vi "Basic.vi"() -> ()   [LabVIEW 2022 SP3, in "GettingStarted_5774_Host.lvlib"]
uses:
  GettingStarted_5774_Host.lvlib
  <vilib>/userDefined/High Color/nirio_resource_hc.ctl
  <instrlib>/FlexRIO/API/Host/v1/NI FlexRIO/API/Reference Clock Source.ctl
  <vilib>/FPGAPlugInAG/PXIe-5774 (KU060)/niLvFpga_Open_PXIe-5774 (KU060).vi
  <vilib>/rvi/interface/common/dynamic/niFpgaDynamicAddResources.vi
  <instrlib>/FlexRIO/API/Host/v1/NI FlexRIO/API/Configure Reference Clock.vi
  <instrlib>/FlexRIO/API/Host/v1/NI FlexRIO/API/Get Property Reference - Fpga Small.vi
  <instrlib>/FlexRIO/API/Host/v1/NI FlexRIO/API/Configure Analog Start Trigger.vi
  <instrlib>/FlexRIO/API/Host/v1/NI FlexRIO/API/Configure Digital Edge Start Trigger.vi
  <instrlib>/FlexRIO/API/Host/v1/NI FlexRIO/API/Configure Immediate Start Trigger.vi
  <instrlib>/FlexRIO/API/Host/v1/NI FlexRIO/API/Read Stream 1D WDT.vi
  <vilib>/measure/maspectr.llb/FFT Power Spectrum and PSD for N Chan.vi
  <vilib>/Utility/error.llb/Error Cluster From Error Code.vi
  <vilib>/rvi/errors/niLvFpgaAdjustHostInterfaceError.vi
  <vilib>/FPGAPlugInAG/Dynamic/niLvFpga_Close_Dynamic.vi
  <vilib>/rvi/interface/nirviOpenFPGA/nirviOpenFPGA.xnode
  FPGA Bitfiles/PXIe_5774_KU060.lvbitx
  <vilib>/rvi/interface/nirviReadWriteControl/nirviReadWriteControl.xnode
  <vilib>/rvi/interface/nirviCloseFPGA/nirviCloseFPGA.xnode
  <instrlib>/FlexRIO/API/Host/v1/NI FlexRIO API v1.lvlib
  <resource>/objmgr/niflexrioapiStream.rc
  <vilib>/measure/NI_MAPro.lvlib
  <resource>/objmgr/niflexrioapiChannel.rc
  NiFpgaLv.dll
  <vilib>/rvi/interface/Simulation/niFpgaSimulationCallBeginRW.vi
panel:
  in  "Threshold":i16
  out "HighValue":bool
  in  "reference clock source":T1 items=["Default", "Onboard", "PXI_Clk10", "External", "None", "Baseboard Reference"]
  in  "AI1 Range":dbl(ring)=1.0 items=["1V"=1.0, "200mV"=0.2]
  in  "AI0 Range":dbl(ring)=1.0 items=["1V"=1.0, "200mV"=0.2]
  in  "AI1 Offset (V)":dbl
  in  "AI0 Offset (V)":dbl
  out "Sample Rate":dbl=3200000000.0 format="%#_6p"
  in  "ADC Interleaving Factor":i32=1 min=0 max=2 step=1
  in  "AI num samples":u64=320 step=16
  in  "AI channels":string="AI0,AI1"
  out "Device Power":dbl(slide) scale=-1.0..38.0 scale format="%#_3p"
  out "FPGA Temperature":dbl(slide) scale=0.0..100.0 scale format="%#_3p"
  in  "Trigger Type":enum32{"Immediate", "Analog", "Digital"}(tab)
  in  "trigger channel":string(combo)="AI0"
  in  "rising edge?":bool=TRUE
  in  "level (V)":dbl format="%#_3p"
  in  "hysteresis (V)":dbl format="%#_3p"
  in  "digital trigger source":string(combo)
  in  "stop":bool
  in  "Waveform Tab Control":enum32{"AI Time Domain", "AI Frequency Domain"}(tab)
  out "Waveform Graph":waveform(dbl)[](graph)
  out "FFT":cluster{"f0":dbl, "df":dbl, "magnitude":dbl[]}[](graph) caption="Waveform Graph"
  out "error out":errorcluster
  out "Limit (W)":dbl
  out "Power (W)":dbl
  out "Limit (C)":dbl
  out "Temp (C)":dbl format="%#_4p"
  in  "RIO Device":T2
  # "Overview: Configure an acquisition for a FlexRIO target and transfer the data to the host using the FlexRIO Host API.  Loop an output waveform\nRequirements: FlexRIO\nInstructions: \n 1. Select the RIO Device that corresponds to the FlexRIO target. \n 2. Optionally configure the clocking, stream, and trigger. \n 3. Run the VI"
  # "Resource Configuration"
  # "Clocking configuration"
  # "Input Waveform Configuration"
  # "Device Monitoring"
  # "Modified:\nDevice Utilization\n---------------------------\nTotal Slices: 41.3% (17139 out of 41460)\nSlice Registers: 15.5% (102931 out of 663360)\nSlice LUTs: 25.5% (84631 out of 331680)\nBlock RAMs: 23.0% (248 out of 1080)\nDSP48s: 0.2% (6 out of 2760)"
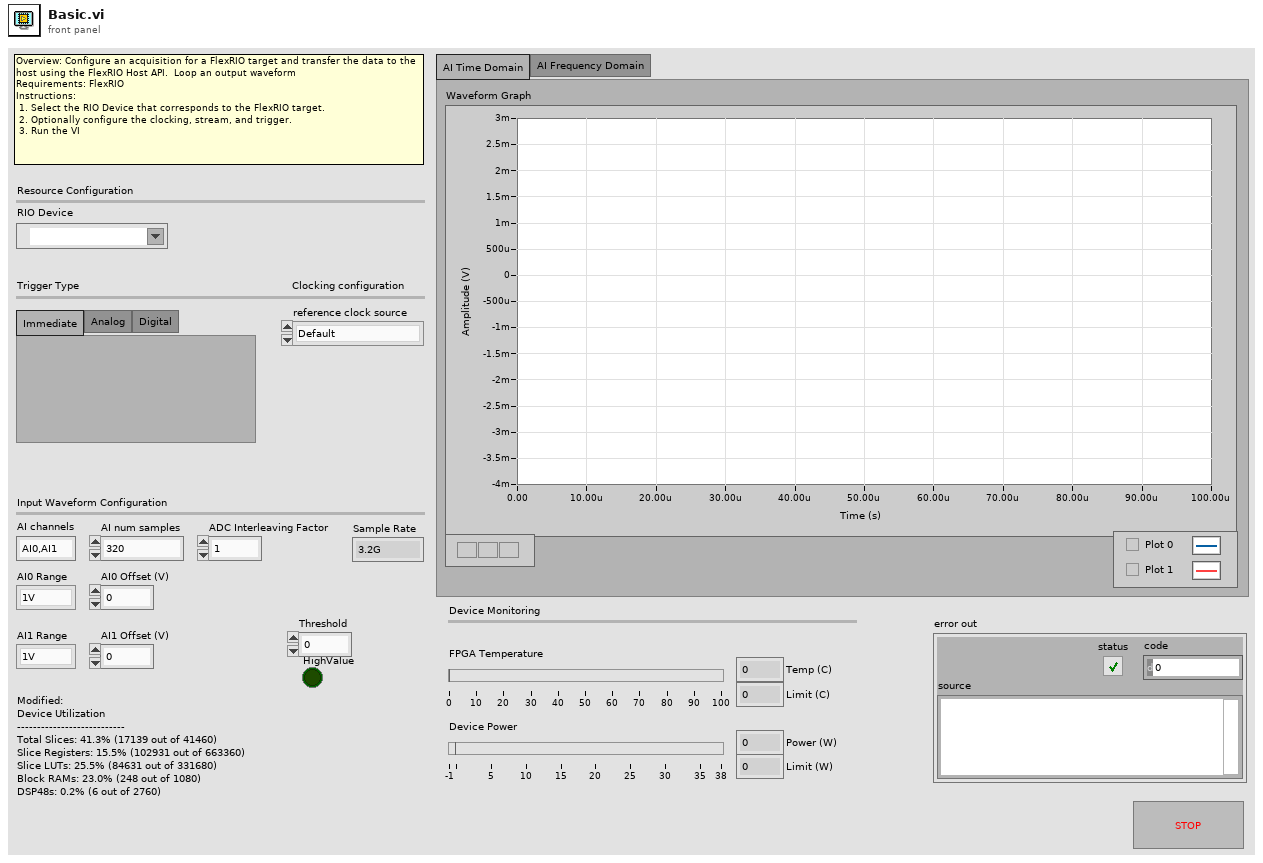
[diagram p1: front panel]
types:
  T1 = typedef "NI FlexRIO API v1.lvlib/Reference Clock Source.ctl" = i32
  T2 = typedef "nirio_resource_hc.ctl" = tag
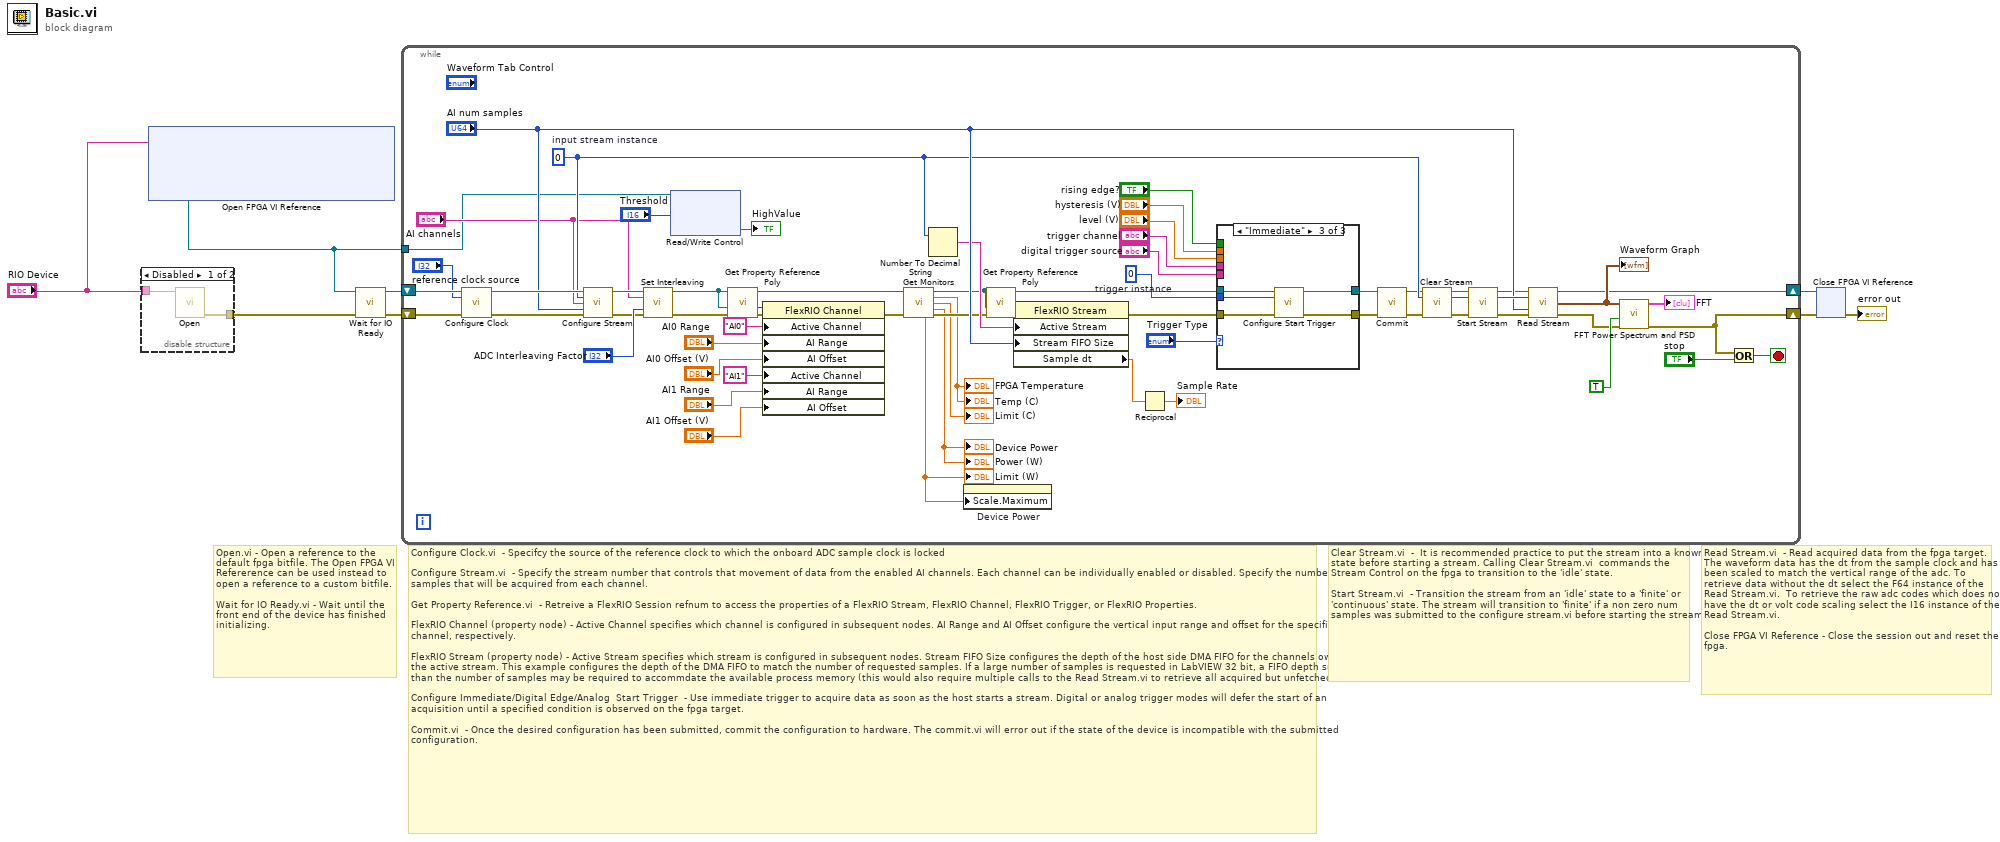
[diagram p0: block diagram]
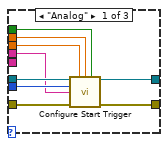
[diagram p3: hidden frame]
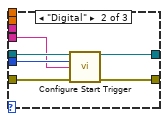
[diagram p4: hidden frame]
diagram:
  # "Read Stream.vi  - Read acquired data from the fpga target. The waveform data has the dt from the sample clock and has been scaled to match the vertical range of the adc. To retrieve data without the dt select the F64 instance of the Read Stream.vi.  To retrieve the raw adc codes which does not have the dt or volt code scaling select the I16 instance of the Read Stream.vi.  \n\nClose FPGA VI Reference - Close the session out and reset the fpga."
  # "Clear Stream.vi  -  It is recommended practice to put the stream into a known state before starting a stream. Calling Clear Stream.vi  commands the Stream Control on the fpga to transition to the 'idle' state.\n\nStart Stream.vi  - Transition the stream from an 'idle' state to a 'finite' or 'continuous' state. The stream will transition to 'finite' if a non zero num samples was submitted to the configure stream.vi before starting the stream."
  # "Configure Clock.vi  - Specifcy the source of the reference clock to which the onboard ADC sample clock is locked\n\nConfigure Stream.vi  - Specify the stream number that controls that movement of data from the enabled AI channels. Each channel can be individually enabled or disabled. Specify the number of samples that will be acquired from each channel. \n\nGet Property Reference.vi  - Retreive a FlexRIO Session refnum to access the properties of a FlexRIO Stream, FlexRIO Channel, FlexRIO Trigger, or FlexRIO Properties.\n\nFlexRIO Channel (property node) - Active Channel specifies which channel is configured in subsequent nodes. AI Range and AI Offset configure the vertical input range and offset for the specified channel, respectively.\n\nFlexRIO Stream (property node) - Active Stream specifies which stream is configured in subsequent nodes. Stream FIFO Size configures the depth of the host side DMA FIFO for the channels owned by the active stream. This example configures the depth of the DMA FIFO to match the number of requested samples. If a large number of samples is requested in LabVIEW 32 bit, a FIFO depth smaller than the number of samples may be required to accommdate the available process memory (this would also require multiple calls to the Read Stream.vi to retrieve all acquired but unfetched data). \n\nConfigure Immediate/Digital Edge/Analog  Start Trigger  - Use immediate trigger to acquire data as soon as the host starts a stream. Digital or analog trigger modes will defer the start of an acquisition until a specified condition is observed on the fpga target. \n\nCommit.vi  - Once the desired configuration has been submitted, commit the configuration to hardware. The commit.vi will error out if the state of the device is incompatible with the submitted configuration."
  # "Open.vi - Open a reference to the default fpga bitfile. The Open FPGA VI Refererence can be used instead to open a reference to a custom bitfile.\n\nWait for IO Ready.vi - Wait until the front end of the device has finished initializing."
  n1 = disable-structure shown="Disabled" {
    disable-tunnel: [w10 _] -> w5
    disable-tunnel: "RIO Device" -> [w9 _]
    frame Disabled {
      n2 = call <instrlib>:"Open.vi"("RIO Device"=w9) -> ("error out"=w10:errorcluster)  [unwired: 13 in, 1 out]
    }
    frame Enabled {
    }
  }
  n3 = xnode "Open FPGA VI Reference"("resource name"="RIO Device") -> ("FPGA VI Reference Out"=w1:refnum<k20>)  [unwired: 1 in, 1 out]
  n4 = call <instrlib>:"Wait for IO Ready.vi"("fpga interface in"=w1, "error in"=w5) -> ("fpga interface out"=w6:refnum<k20>, "error out"=w7:errorcluster)  [unwired: 10 in, 2 out]
  n5 = while {
    shift-right: [w43] -> w3
    shift-left: w7 -> [w58]
    shift-right: [w49] -> w4
    shift-left: w6 -> [w57]
    tunnel: w1 -> [w13]
    stop <- w45 stop-if-true
    w59 = u32 0  # trigger instance
    w48 = u32 0  # input stream instance
    n6 = call-poly <instrlib>:"Configure Clock.vi"("fpga interface in"=w57, "reference clock source"="reference clock source", "error in"=w58) -> ("fpga interface out"=w65:refnum<k20>, "error out"=w64:errorcluster)  [unwired: 11 in]
    n7 = call <instrlib>:"Configure Stream.vi"("fpga interface in"=w65, "stream instance"=w48, "channels enabled"="AI channels", "num samples"="AI num samples", "error in"=w64) -> ("fpga interface out"=w41:refnum<k20>, "error out"=w40:errorcluster)  [unwired: 7 in, 2 out]
    n8 = call "Set Interleaving.vi"("fpga interface in"=w41, "AI channels enabled"="AI channels", "ADC Interleaving Factor"="ADC Interleaving Factor", "error in (no error)"=w40) -> ("fpga interface out"=w15:refnum<k20>, "error out"=w19:errorcluster)  [unwired: 10 in]
    n9 = xnode "Read/Write Control"("FPGA VI Reference In"=w13, "Threshold"="Threshold") -> ("HighValue"=→"HighValue":bool)  [unwired: 1 in, 2 out]
    n10 = call-poly <instrlib>:"Get Property Reference Poly.vi"("error in (no error)"=w19, "fpga interface in"=w15) -> ("error out"=w22:errorcluster, "property reference"=w23:refnum<k20>)  [unwired: 4 in, 1 out]
    n11 = property class="FlexRIO Channel"(reference=w23, error in=w22, "Active Channel"="AI0" ("Active Stream"), "AI Range"="AI0 Range", "AI Offset"="AI0 Offset (V)", "Active Channel"="AI1" ("Active Stream"), "AI Range"="AI1 Range", "AI Offset"="AI1 Offset (V)") -> (error out=w18:errorcluster)  [unwired: 1 out]
    n12 = call "Get Monitors.vi"("fpga interface in"=w15, "error in (no error)"=w18) -> ("fpga interface out"=w36:refnum<k20>, "FPGA Temperature (C)"=→"Temp (C)" →"FPGA Temperature":dbl, "Temperature Limit (C)"=→"Limit (C)":dbl, "Total Power (W)"=→"Power (W)" →"Device Power":dbl, "Power Limit (W)"=w32:dbl, "error out"=w39:errorcluster)  [unwired: 8 in]
    "Limit (W)" <- w32
    n13 = Number To Decimal String(number=w48) -> (decimal integer string=w61:string)  [unwired: 1 in]
    n14 = property on="Device Power" class="Slide (strict)"("Scale.Maximum"=w32) -> ()  [unwired: 2 in, 2 out]
    n15 = call-poly <instrlib>:"Get Property Reference Poly.vi"("error in (no error)"=w39, "fpga interface in"=w36) -> ("error out"=w38:errorcluster, "property reference"=w37:refnum<k20>)  [unwired: 4 in, 1 out]
    n16 = property class="FlexRIO Stream"(reference=w37, error in=w38, "Active Stream"=w61, "Stream FIFO Size"="AI num samples") -> (error out=w52:errorcluster, "Sample dt"=w47:dbl)  [unwired: 1 out]
    n17 = Reciprocal(x=w47) -> (1/x=→"Sample Rate":dbl)
    n18 = case shown="\"Immediate\"" "Trigger Type" {
      tunnel: w36 -> [w81 w87 w92]
      tunnel: w52 -> [w80 w86 w91]
      tunnel: [w79 w85 w90] -> w29
      tunnel: [w78 w84 w89] -> w30
      tunnel: w59 -> [w77 w83 w88]
      tunnel: "trigger channel" -> [w76 _ _]
      tunnel: "level (V)" -> [w75 _ _]
      tunnel: "hysteresis (V)" -> [w74 _ _]
      tunnel: "rising edge?" -> [w73 _ _]
      tunnel: "digital trigger source" -> [_ w82 _]
      frame "Analog" {
        n19 = call-poly <instrlib>:"Configure Start Trigger.vi"("fpga interface in"=w81, "level"=w75, "hysteresis"=w74, "rising edge?"=w73, "trigger instance"=w77, "channel"=w76, "error in"=w80) -> ("fpga interface out"=w79:refnum<k20>, "error out"=w78:errorcluster)  [unwired: 6 in, 1 out]
      }
      frame "Digital" {
        n20 = call-poly <instrlib>:"Configure Start Trigger.vi"("fpga interface in"=w87, "trigger instance"=w83, "trigger source"=w82, "error in"=w86) -> ("fpga interface out"=w85:refnum<k20>, "error out"=w84:errorcluster)  [unwired: 9 in, 1 out]
      }
      frame "Immediate" {
        n21 = call-poly <instrlib>:"Configure Start Trigger.vi"("fpga interface in"=w92, "trigger instance"=w88, "error in"=w91) -> ("fpga interface out"=w90:refnum<k20>, "error out"=w89:errorcluster)  [unwired: 10 in, 1 out]
      }
    }
    n22 = call <instrlib>:"Commit.vi"("fpga interface in"=w29, "error in"=w30) -> ("fpga interface out"=w26:refnum<k20>, "error out"=w27:errorcluster)  [unwired: 12 in]
    n23 = call <instrlib>:"Clear Stream.vi"("fpga interface in"=w26, "stream instance"=w48, "error in"=w27) -> ("fpga interface out"=w68:refnum<k20>, "stream instance out"=w67:u32, "error out"=w66:errorcluster)  [unwired: 10 in]
    n24 = call <instrlib>:"Start Stream.vi"("fpga interface in"=w68, "stream instance"=w67, "error in"=w66) -> ("fpga interface out"=w51:refnum<k20>, "stream instance out"=w63:u32, "error out"=w50:errorcluster)  [unwired: 10 in]
    n25 = call-poly <instrlib>:"Read Stream.vi"("fpga interface in"=w51, "stream instance"=w63, "samples"="AI num samples", "error in"=w50) -> ("fpga interface out"=w49:refnum<k20>, "read data"=w54:waveform(dbl)[], "error out"=w44:errorcluster)  [unwired: 7 in, 2 out]
    "Waveform Graph" <- w54
    n26 = call-poly <vilib>:"FFT Power Spectrum and PSD.vi"("error in (no error)"=w44, "dB On (F)"=TRUE, "time signals"=w54) -> ("error out"=w43:errorcluster, "Power Spectrum / PSD"=→"FFT":cluster{"f0":dbl, "df":dbl, "magnitude":dbl[]}[])  [unwired: 5 in, 2 out]
    n27 = Or(x=w43, y="stop") -> (x .or. y?=w45:bool)
  }
  n28 = xnode "Close FPGA VI Reference"("FPGA VI Reference In"=w4, "error in"=w3) -> ("error out"=→"error out":errorcluster)
